vi "Execute Default event.vi"(6 "Module ID":i32, 8 "error in":errorcluster, 9 "Event":string, 10 "Library":refnum<class "Library.lvclass">, 11 "Project":refnum<class "Project.lvclass">) -> (0 "error out":errorcluster)   [LabVIEW 2020, in "Panther Dashboard.lvlib"]
doc: "This VI checks the Main.vi State of the selected DQMH Module"
uses:
  Panther Dashboard.lvlib
  Class/Project/Project.lvclass
  Class/Library/Library.lvclass
  Class/Project/Project.lvclass/Project.ctl
  Class/Library/Library.lvclass/Library.ctl
  Class/Library/Read Type.vi
  Class/Library/Read Library Ref.vi
  Class/Project/Read Main App Inst Ref.vi
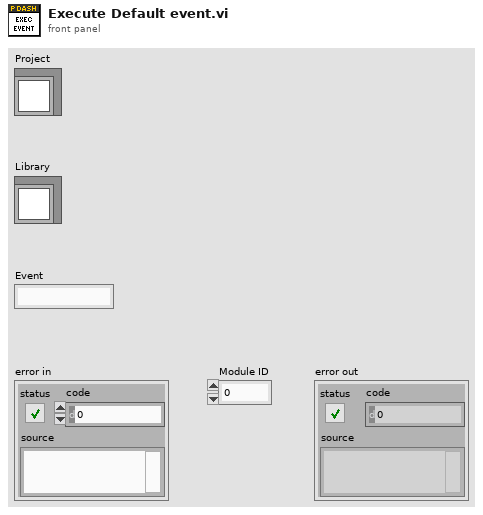
[diagram p1: front panel]
types:
  T1 = typedef "Panther Dashboard.lvlib/Module type--enum.ctl" = enum16{"Singleton", "Cloneable"}
  T2 = enum32{"Bad", "Idle", "Run top level", "Running"}
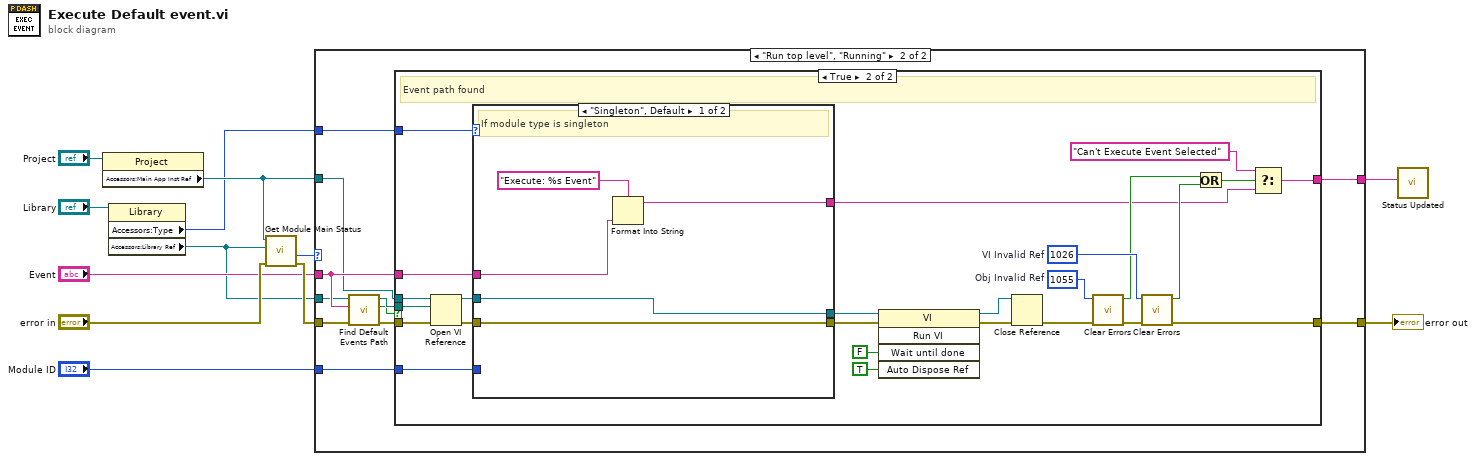
[diagram p0: block diagram]
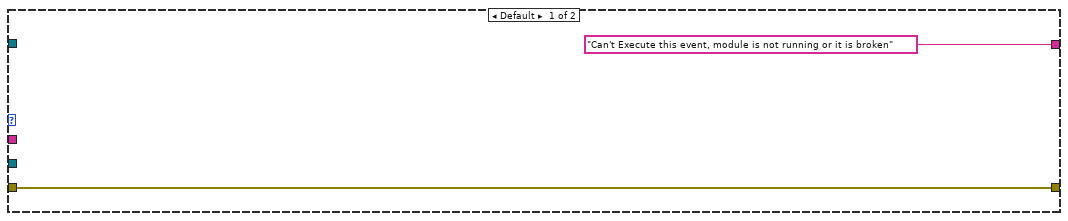
[diagram p2: hidden frame]
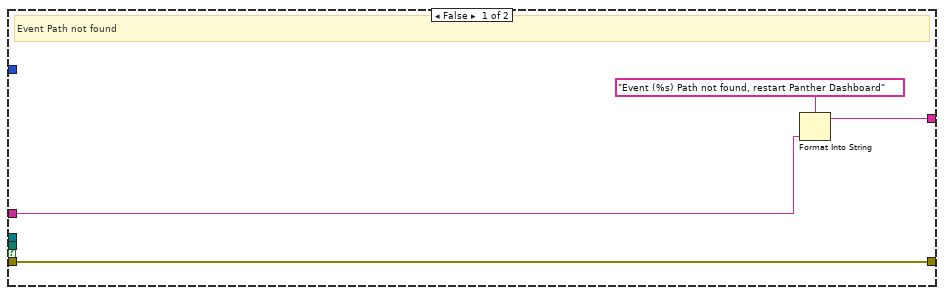
[diagram p3: hidden frame]
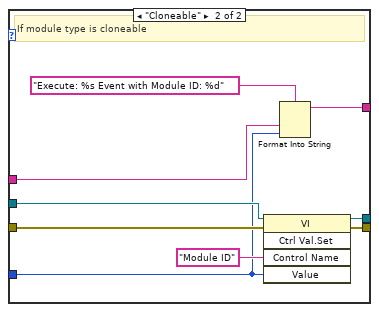
[diagram p4: hidden frame]
diagram:
  n1 = property class="Project"(reference="Project") -> ("Accessors:Main App Inst Ref"=w4:refnum<vi>)  [unwired: 1 in, 2 out]
  n2 = property class="Library"(reference="Library") -> ("Accessors:Type"=w1:T1, "Accessors:Library Ref"=w2:refnum<vi>)  [unwired: 1 in, 2 out]
  n3 = call "Get Module Main Status.vi"("error in"="error in", "Library in"=w2, "application Instance"=w4) -> ("error out"=w11:errorcluster, "Module Exec State"=w6:T2)  [unwired: 6 in, 1 out]
  n4 = case shown="\"Run top level\", \"Running\"" w6 {
    tunnel: w11 -> [w14 w25]
    tunnel: [w14 w23] -> w12
    tunnel: w1 -> [_ w21]
    tunnel: "Module ID" -> [_ w20]
    tunnel: "Event" -> [_ w19]
    tunnel: ["Can't Execute this event, module is not running or it is broken" ("t") w18] -> w7
    tunnel: w4 -> [_ w17]
    tunnel: w2 -> [_ w16]
    frame Default {
    }
    frame "Run top level", "Running" {
      n5 = call "Find Default Events Path.vi"("error in"=w25, "Event"=w19, "DQMH Library Ref"=w16) -> ("error out"=w24:errorcluster, "Event Path Found?"=w15:bool, "Event Path"=w22:path)  [unwired: 6 in]
      n6 = case shown="True" w15 {
        tunnel: w24 -> [w29 w54]
        tunnel: [w29 w52] -> w23
        tunnel: w22 -> [_ w47]
        tunnel: w21 -> [_ w44]
        tunnel: w20 -> [_ w42]
        tunnel: w19 -> [w27 w38]
        tunnel: [w28 w33] -> w18
        tunnel: w17 -> [_ w30]
        frame False {
          # "Event Path not found"
          n7 = Format Into String(format string="Event (%s) Path not found, restart Panther Dashboard", w27) -> (resulting string=w28:string)  [unwired: 2 in, 1 out]
        }
        frame True {
          w46 = 1055  # Obj Invalid Ref
          w45 = 1026  # VI Invalid Ref
          # "Event path found"
          n8 = Open VI Reference(application reference (local)=w30, vi path=w47, error in (no error)=w54) -> (vi reference=w41:refnum<vi>, error out=w51:errorcluster)  [unwired: 3 in]
          n9 = case shown="\"Singleton\", Default" w44 {
            tunnel: w41 -> [w58 w65]
            tunnel: w51 -> [w59 w67]
            tunnel: [w58 w64] -> w43
            tunnel: [w59 w68] -> w50
            tunnel: w42 -> [_ w62]
            tunnel: w38 -> [w56 w63]
            tunnel: [w55 w61] -> w34
            frame "Singleton", Default {
              # "If module type is singleton"
              n10 = Format Into String(format string="Execute: %s Event", w56) -> (resulting string=w55:string)  [unwired: 2 in, 1 out]
            }
            frame "Cloneable" {
              # "If module type is cloneable"
              n11 = invoke class="VI" method="Ctrl Val.Set"(reference=w65, error in=w67, "Control Name"="Module ID", "Value"=w62) -> (reference out=w64:refnum<vi>, error out=w68:errorcluster)  [unwired: 1 in, 3 out]
              n12 = Format Into String(format string="Execute: %s Event with Module ID: %d", w63, w62) -> (resulting string=w61:string)  [unwired: 2 in, 1 out]
            }
          }
          n13 = invoke class="VI" method="Run VI"(reference=w43, error in=w50, "Wait until done"=FALSE ("Wait Until Done"), "Auto Dispose Ref"=TRUE ("Auto Dispose Reference")) -> (reference out=w31:refnum<vi>, error out=w49:errorcluster)  [unwired: 1 in, 3 out]
          n14 = Close Reference(reference=w31, error in (no error)=w49) -> (error out=w48:errorcluster)
          n15 = call <vilib>:"Clear Errors.vi"("error in (no error)"=w48, "specific error code to clear (0: all)"=w46) -> ("error out"=w53:errorcluster, "specific error cleared?"=w36:bool)  [unwired: 4 in]
          n16 = call <vilib>:"Clear Errors.vi"("error in (no error)"=w53, "specific error code to clear (0: all)"=w45) -> ("error out"=w52:errorcluster, "specific error cleared?"=w37:bool)  [unwired: 4 in]
          n17 = Or(x=w36, y=w37) -> (x .or. y?=w35:bool)
          n18 = Select(t="Can't Execute Event Selected", s=w35, f=w34) -> (s? t:f=w33:string)
        }
      }
    }
  }
  "error out" <- w12
  n19 = call "Status Updated.vi"("Status"=w7) -> ()  [unwired: 10 in, 1 out]
